vi "RDS Child Receive Message.vi"(8 "error in (no error)":errorcluster, 10 "RDS Message":refnum<class "RDS Message.lvclass">, 11 "MCB Instrument in":refnum<class "MCB Instrument.lvclass">) -> (0 "error out":errorcluster, 3 "MCB Instrument out":refnum<class "MCB Instrument.lvclass">)   [LabVIEW 2015, in "MCB Instrument.lvlib" / "MCB Instrument.lvclass"]
uses:
  MCB Instrument.lvclass
  Libraries/RDS Framework/RDS Message Class/RDS Message.lvclass
  Libraries/RDS Framework/RDS Message Class/RDS Message.lvclass/RDS Message.ctl
  Libraries/RDS Child Messages/MCB/MCB Command Message/MCB Command.lvclass
  Libraries/RDS Child Messages/MCB/MCB Command Message/MCB Command.lvclass/MCB Command.ctl
  MCB Instrument.lvclass/MCB Instrument.ctl
  Libraries/RDS Serial Handler/RDS Serial Frame.lvclass/RDS Serial Frame.ctl
  Libraries/RDS Serial Handler/RDS Serial Frame.lvclass
  Actors/RDS Serial Instrument Actor/RDS Serial Instrument Actor.lvclass
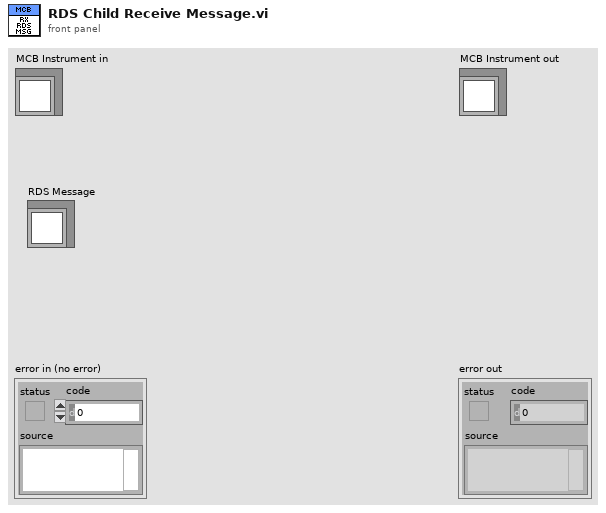
[diagram p1: front panel]
types:
  T1 = typedef "RDS Child Messages.lvlib/RDS Message ID.ctl" = enum16{"RDS Hello World", "String Message", "AIP_Status", "AIP_Command", "GPS_Data", "MCB_Command", "MCB_Status", "Compass_Data", "Depth_Data", "Battery_Data", "Contoller_State", "Set_Mag_Dev", "BTB_Shutdown", "State_Sample_Request", "State_Sample", "PID_Gains_Set", "Helm_Limiter_Set", "Helm_Heading_Command", "Helm_Steering_Command", "Helm_Status", "Controller_Message", "AIP_Set_Min_Depth", "Mission_Controller_State", "Mission_Upload", "Mission_Set_Op_and_Run", "Mission_Settings_Set"}
  T2 = typedef "RDS Child Messages.lvlib/MCB Channel.ctl" = enum16{"PORT", "STBD"}
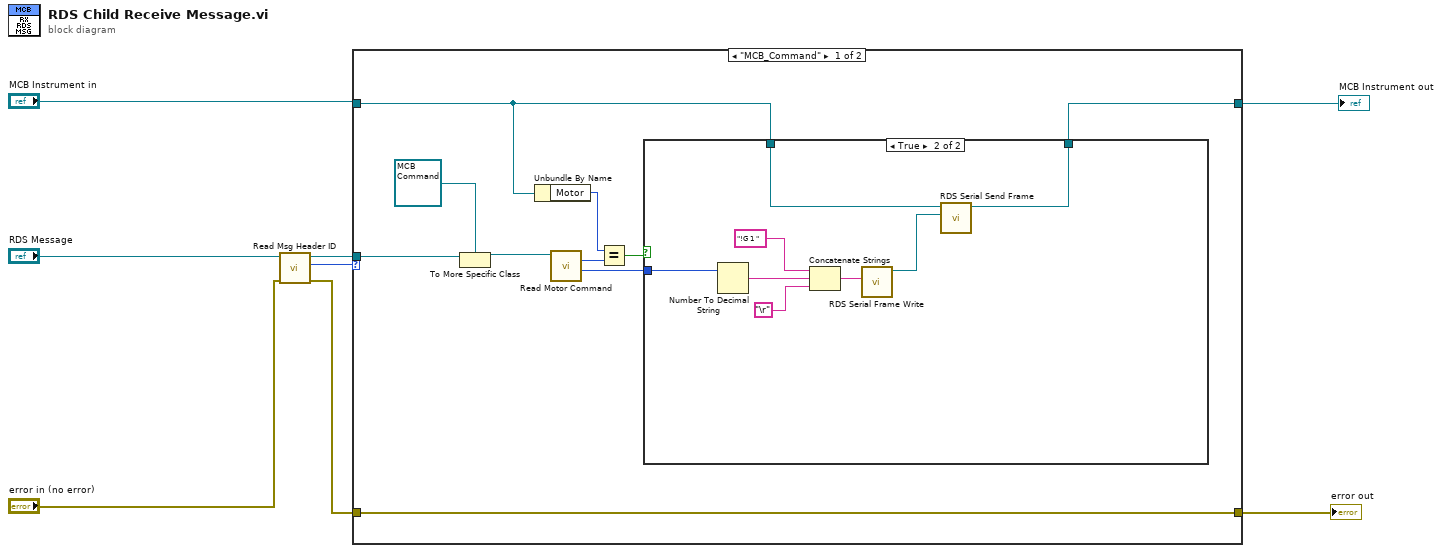
[diagram p0: block diagram]
diagram:
  n1 = call "Read Msg Header ID.vi"("error in (no error)"="error in (no error)", "RDS Message in"="RDS Message") -> ("error out"=w6:errorcluster, "Msg ID"=w8:T1, "RDS Message out"=w7:refnum<class "RDS Message.lvclass">)  [unwired: 5 in, 2 out]
  n2 = case shown="\"MCB_Command\"" w8 {
    tunnel: "MCB Instrument in" -> [w12 w29]
    tunnel: w7 -> [w17 _]
    tunnel: [w16 w29] -> w2
    tunnel: w6 -> [w18 w28]
    tunnel: [w18 w28] -> w1
    frame "MCB_Command" {
      n3 = To More Specific Class(target class=refnum<class "MCB Command.lvclass"> refnum ("RDS Child Messages.lvlib:MCB Command.lvclass"), reference=w17) -> (specific class reference=w14:refnum<class "MCB Command.lvclass">)  [unwired: 1 in, 1 out]
      n4 = Unbundle By Name(w12) -> ("Motor"=w11:T2)
      n5 = call "Read Motor Command.vi"("MCB Command in"=w14) -> ("Motor Command"=w9:i16, "Motor"=w13:T2)  [unwired: 7 in, 2 out]
      n6 = Equal?(x=w11, y=w13) -> (x = y?=w10:bool)
      n7 = case shown="True" w10 {
        tunnel: [w19 w27] -> w16
        tunnel: w12 -> [w19 w26]
        tunnel: w9 -> [_ w23]
        frame False {
        }
        frame True {
          n8 = Number To Decimal String(number=w23) -> (decimal integer string=w22:string)  [unwired: 1 in]
          n9 = Concatenate Strings("!G 1 " ("Serial String"), w22, "\r") -> (w21:string)
          n10 = call "RDS Serial Frame Write.vi"("Serial String"=w21) -> ("RDS Serial Frame out"=w25:refnum<class "RDS Serial Frame.lvclass">)  [unwired: 9 in, 1 out]
          n11 = call "RDS Serial Send Frame.vi"("RDS Frame"=w25, "RDS Serial Instrument Actor in"=w26) -> ("RDS Serial Instrument Actor out"=w27:refnum<class "MCB Instrument.lvclass">)  [unwired: 8 in, 1 out]
        }
      }
    }
    frame "String Message", Default {
    }
  }
  "error out" <- w1
  "MCB Instrument out" <- w2
